vi "Message.vi"(8 "error in (no error)":errorcluster, 9 "Data":variant, 10 "Command":string, 11 "MessageEvent":refnum<user-event>) -> (0 "error out":errorcluster)   [LabVIEW 2019, in "SLL Message.lvlib"]
uses:
  SLL Message.lvlib
  Typedefs/Message.ctl
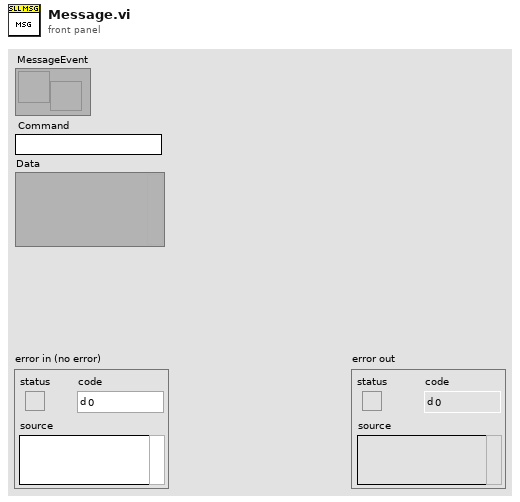
[diagram p1: front panel]
types:
  T1 = typedef "SLL Message.lvlib/Message.ctl" = cluster{"Command":string, "Data":variant, "Fetch Response?":bool, "Response":refnum<notifier>}
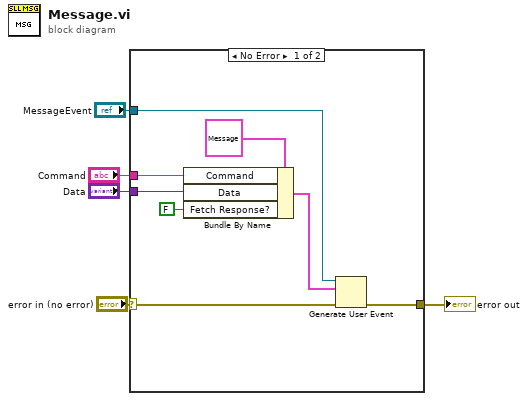
[diagram p0: block diagram]
diagram:
  n1 = case shown="No Error" "error in (no error)" {
    selector: "error in (no error)" -> [w13 w14]
    tunnel: [w12 w14] -> w4
    tunnel: "MessageEvent" -> [w11 _]
    tunnel: "Command" -> [w8 _]
    tunnel: "Data" -> [w7 _]
    frame No Error {
      n2 = Bundle By Name(cluster=T1 {"Command"="", "Data"=variant, "Fetch Response?"=FALSE, "Response"=refnum} ("event data"), "Command"=w8, "Data"=w7, "Fetch Response?"=FALSE) -> (w9:T1)
      n3 = Generate User Event(user event=w11, event data cluster=w9, error in=w13) -> (error out=w12:errorcluster)  [unwired: 1 in, 1 out]
    }
    frame Error {
    }
  }
  "error out" <- w4
